vi "SMBus Process Call.vi"(1 "PEC":u8, 4 "pReadData":u16, 5 "WriteData":u16, 6 "CommandCode":u8, 7 "SlaveAddr":u8, 9 "SMBUSIndex":i32, 10 "DevIndex":i32, 11 "DevType":i32) -> (2 "function return":i32, 3 "pReadData out":u16)   [LabVIEW 2010, in "ControlSMBus.lvlib"]
doc: "int WINAPI SMBus_ProcessCall(int DevType,int DevIndex,int SMBUSIndex,unsigned char SlaveAddr,unsigned char CommandCode,unsigned short WriteData, unsigned short *pReadData,unsigned char PEC);"
uses:
  ControlSMBus.lvlib
  ControlSMBus/Ginkgo_Driver.dll
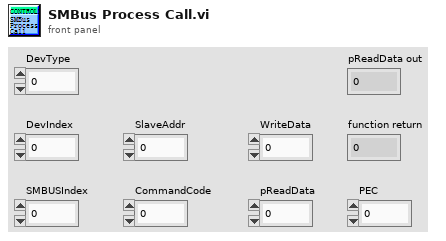
[diagram p1: front panel]
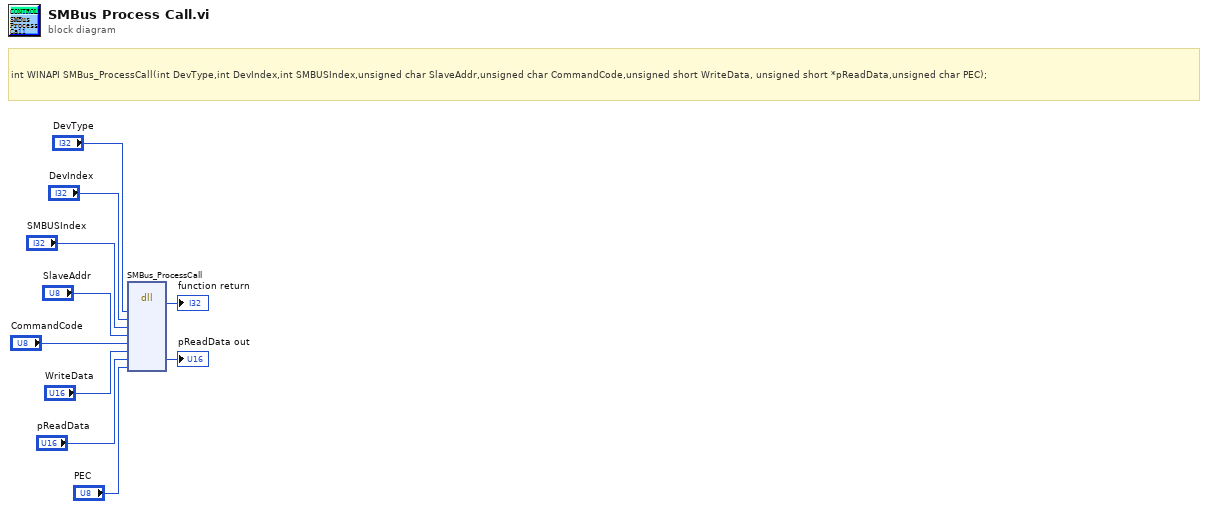
[diagram p0: block diagram]
diagram:
  # "int WINAPI SMBus_ProcessCall(int DevType,int DevIndex,int SMBUSIndex,unsigned char SlaveAddr,unsigned char CommandCode,unsigned short WriteData, unsigned short *pReadData,unsigned char PEC);"
  n1 = dll-call lib="E:/Project/vt_ginkgo/truck/Ginkgo Driver/vs2010/Ginkgo_USB-I2C&SPI&CAN_API_v2.0.3.3/lib/labview_32bit/ControlSMBus/Ginkgo_Driver.*" fn="SMBus_ProcessCall"("DevType"="DevType", "DevIndex"="DevIndex", "SMBUSIndex"="SMBUSIndex", "SlaveAddr"="SlaveAddr", "CommandCode"="CommandCode", "WriteData"="WriteData", "pReadData"="pReadData", "PEC"="PEC") -> (→"function return":i32, "pReadData"=→"pReadData out":u16)  [unwired: 10 in, 2 out]
